vi "kPIDsat.vi"(8 "PID Gains":cluster{"Kp":dbl, "Kd":dbl, "Ki":dbl}, 9 "Sat Limit":dbl, 10 "Position":dbl, 11 "Reference":dbl) -> (3 "Control":dbl)   [LabVIEW 2016, in "KevLib01.lvlib"]
uses:
  KevLib01.lvlib
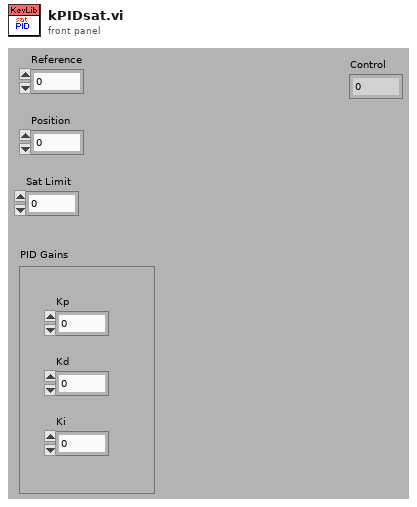
[diagram p1: front panel]
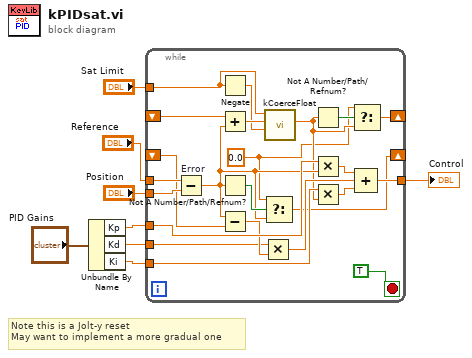
[diagram p0: block diagram]
diagram:
  # "Note this is a Jolt-y reset\nMay want to implement a more gradual one"
  n1 = Unbundle By Name("PID Gains") -> ("Kp"=w4:dbl, "Kd"=w3:dbl, "Ki"=w2:dbl)
  n2 = while {
    tunnel: w4 -> [w30]
    tunnel: "Reference" -> [w29]
    tunnel: "Position" -> [w28]
    shift-right: [w14] -> _
    shift-left: _ -> [w27]
    tunnel: w3 -> [w25]
    shift-right: [w13] -> _
    shift-left: _ -> [w24]
    tunnel: w2 -> [w23]
    tunnel: [w19] -> w1
    tunnel: "Sat Limit" -> [w17]
    stop <- TRUE stop-if-true
    w9 = 0.0 ("t")
    n3 = Subtract "Error"(x=w29, y=w28) -> (x-y=w12:dbl)
    n4 = Negate(x=w17) -> (-x=w16:dbl)
    n5 = Add(x=w24, y=w12) -> (x+y=w18:dbl)
    n6 = Not A Number/Path/Refnum?(number/path/refnum=w12) -> (NaN/Path/Refnum?=w15:bool)
    n7 = Subtract(x=w12, y=w27) -> (x-y=w26:dbl)
    n8 = Multiply(x=w25, y=w26) -> (x*y=w21:dbl)
    n9 = Select(t=w9, s=w15, f=w12) -> (s? t:f=w14:dbl)
    n10 = call "kCoerceFloat.vi"("lower"=w16, "input"=w18, "upper"=w17) -> ("output"=w10:dbl)  [unwired: 8 out]
    n11 = Not A Number/Path/Refnum?(number/path/refnum=w10) -> (NaN/Path/Refnum?=w11:bool)
    n12 = Multiply(x=w30, y=w12) -> (x*y=w22:dbl)
    n13 = Multiply(x=w23, y=w10) -> (x*y=w20:dbl)
    n14 = Select(t=w9, s=w11, f=w10) -> (s? t:f=w13:dbl)
    n15 = Compound Arithmetic op=ADD(w22, w21, w20) -> (w19:dbl)
  }
  "Control" <- w1
